vi "Webcam timer.vi"(6 "Inc?":bool, 7 "Reset":bool, 8 "error in (no error)":errorcluster) -> (0 "error out":errorcluster, 2 "Int":i32, 3 "Time":dbl)   [LabVIEW 2016]
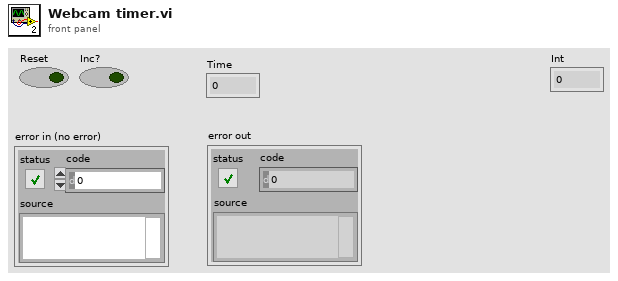
[diagram p1: front panel]
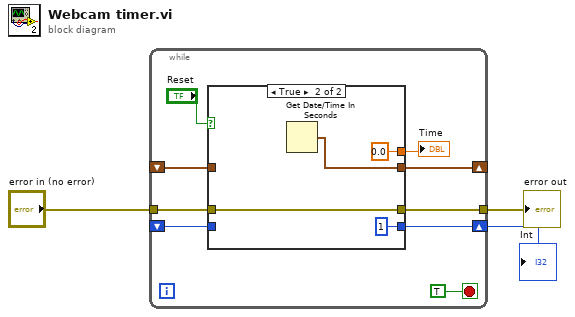
[diagram p0: block diagram]
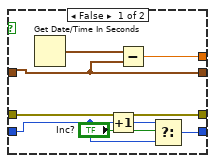
[diagram p2: hidden frame]
diagram:
  n1 = while {
    shift-right: [w11] -> _
    shift-left: _ -> [w9]
    tunnel: "error in (no error)" -> [w7]
    tunnel: [w6] -> w2
    shift-right: [w5] -> w1
    shift-left: _ -> [w4]
    stop <- TRUE stop-if-true
    n2 = case shown="True" "Reset" {
      tunnel: [w19 w24] -> w11
      tunnel: w9 -> [w19 _]
      tunnel: [w18 0.0] -> w8
      tunnel: w7 -> [w17 w22]
      tunnel: [w17 w22] -> w6
      tunnel: [w16 1] -> w5
      tunnel: w4 -> [w14 _]
      frame False {
        n3 = Get Date/Time In Seconds() -> (seconds since 1Jan1904=w20:timestamp)
        n4 = Increment(x=w14) -> (x+1=w15:i32)
        n5 = Subtract(x=w20, y=w19) -> (x-y=w18:dbl)
        n6 = Select(t=w15, s="Inc?", f=w14) -> (s? t:f=w16:i32)
      }
      frame True {
        n7 = Get Date/Time In Seconds() -> (seconds since 1Jan1904=w24:timestamp)
      }
    }
    "Time" <- w8
  }
  "error out" <- w2
  "Int" <- w1
